vi "Write RC Type.vi"(8 "error in (no error)":errorcluster, 10 "RC Type [STM]":T1=enum."STM", 11 "Instrument in":refnum<class "Instrument.lvclass">) -> (0 "error out":errorcluster, 3 "Instrument out":refnum<class "Instrument.lvclass">)   [LabVIEW 2019, in "Instrument.lvclass"]
uses:
  Instrument.lvclass
  RemoteControl/Typedefs/RC Com Type--enum.ctl
  Instrument.lvclass/Instrument.ctl
  RemoteControl/RemoteControl.lvclass
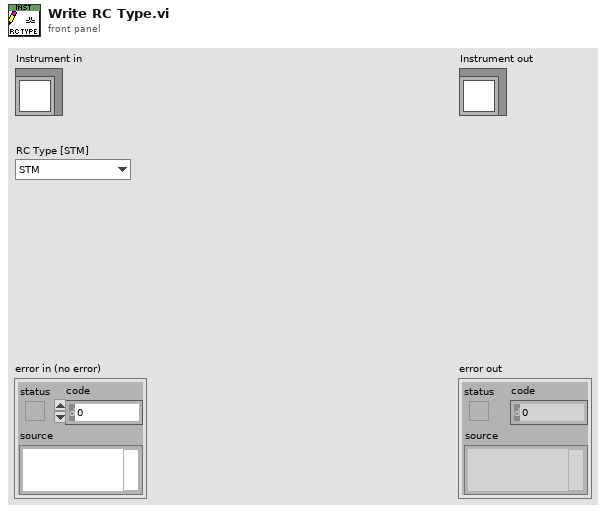
[diagram p1: front panel]
types:
  T1 = typedef "RemoteControl.lvclass/RC Com Type--enum.ctl" = enum16{"RC", "STM", "ZMQ"}
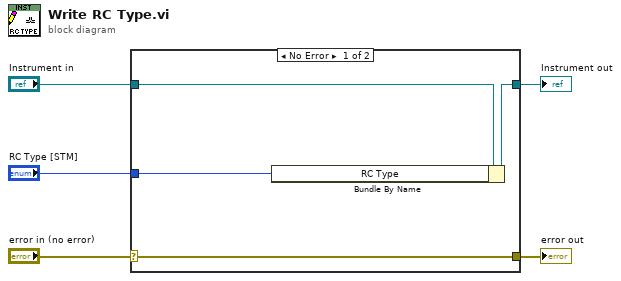
[diagram p0: block diagram]
diagram:
  n1 = case shown="No Error" "error in (no error)" {
    selector: "error in (no error)" -> [w9 w10]
    tunnel: [w9 w10] -> w4
    tunnel: [w7 w11] -> w2
    tunnel: "Instrument in" -> [w8 w11]
    tunnel: "RC Type [STM]" -> [w6 _]
    frame No Error {
      n2 = Bundle By Name(cluster=w8, "RC Type"=w6) -> (w7:refnum<class "Instrument.lvclass">)
    }
    frame Error {
    }
  }
  "error out" <- w4
  "Instrument out" <- w2
